vi "MultiAssertBuild TRef FinderCallback.vi"(4 "context in":variant, 5 "objref":refnum<vi>) -> (1 "context out":variant, 2 "traverse flags":i32)   [LabVIEW 2016]
doc: "This VI is the callback used for Traverse for GObjects.vi. It simply builds up an array of all references that match the specified class name for the traversal."
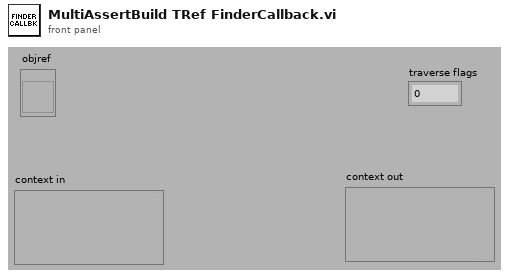
[diagram p1: front panel]
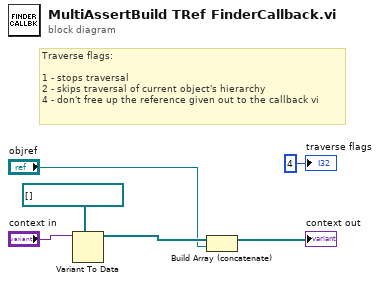
[diagram p0: block diagram]
diagram:
  # "Traverse flags:\n\n1\t- stops traversal \n2\t- skips traversal of current object's hierarchy\n4 - don't free up the reference given out to the callback vi"
  n1 = Variant To Data(type=refnum<vi>[] [], Variant="context in") -> (data=w3:refnum<vi>[])  [unwired: 1 in, 1 out]
  n2 = Build Array (concatenate)(w3, "objref") -> (→"context out":refnum<vi>[])
  "traverse flags" <- 4 ("Traverse Flags")
